vi "Save Settings.vi"(8 "error in":errorcluster, 9 "Head Channel":i16, 10 "Pulsar Handle":i16, 11 "OphirFastX (in)":refnum<k7>) -> (0 "error out":errorcluster, 3 "OphirFastX (out)":refnum<k7>)   [LabVIEW 2009]
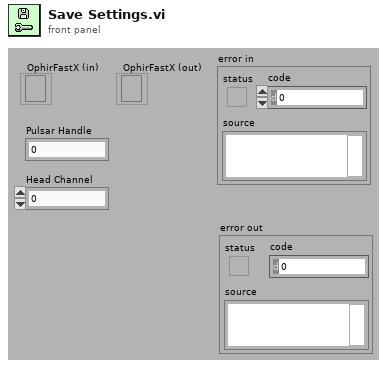
[diagram p1: front panel]
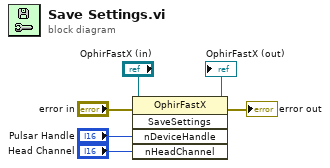
[diagram p0: block diagram]
diagram:
  n1 = invoke class="OphirFastX" method="SaveSettings"(reference="OphirFastX (in)", error in="error in", "nDeviceHandle"="Pulsar Handle", "nHeadChannel"="Head Channel") -> (reference out=→"OphirFastX (out)":refnum<k7>, error out=→"error out":errorcluster)  [unwired: 1 in, 3 out]
